vi "Organize Tidepool List Output.vi"(8 "error in":errorcluster, 11 "dir list":T2[](array[typedef])) -> (0 "error in 2":errorcluster, 3 "Array":T1(array[cluster]))   [LabVIEW 2014]
uses:
  <vilib>/FTP/ftp2.llb/FTP File Info.ctl
  <vilib>/FTP/NI_FTP.lvlib
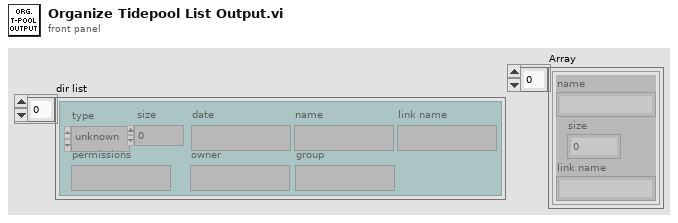
[diagram p1: front panel]
types:
  T1 = cluster{"name":string, "size":i32, "link name":string}[]
  T2 = typedef "NI_FTP.lvlib/FTP File Info.ctl" = cluster{"type":enum16{"unknown", "file", "dir", "link"}, "permissions":string, "owner":string, "group":string, "size":i32, "date":string, "name":string, "link name":string}
  T3 = cluster{"name":string, "size":i32, "name":string}
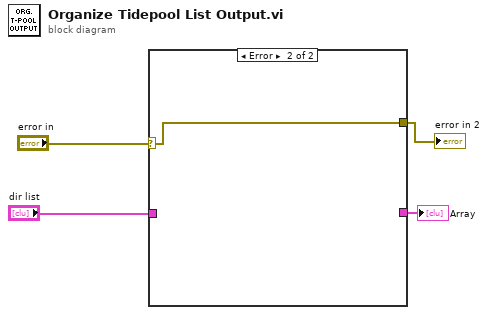
[diagram p0: block diagram]
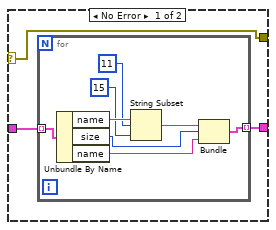
[diagram p2: hidden frame]
diagram:
  n1 = case shown="Error" "error in" {
    selector: "error in" -> [w5 w16]
    tunnel: [w7 _] -> w4
    tunnel: "dir list" -> [w6 _]
    tunnel: [w5 w16] -> w1
    frame No Error {
      n2 = for {
        tunnel: w6 -> [w15] mode=indexing
        tunnel: [w9] -> w7 mode=indexing
        n3 = Unbundle By Name(w15) -> ("name"=w14:string, "size"=w10:i32, "name"=w8:string)
        n4 = String Subset(string=w14, offset (0)=11, length (rest)=15 ("offset (0)")) -> (substring=w11:string)
        n5 = Bundle("name"=w11, "size"=w10, "name"=w8) -> (w9:T3)  [unwired: 1 in]
      }
    }
    frame Error {
    }
  }
  "Array" <- w4
  "error in 2" <- w1
